vi "CircularBuffer.DVRtoRef.vi"(10 "Ref":T1) -> (2 "Ref":u32 format="%08x")   [LabVIEW 2016, in "CircularBuffer.lvclass"]
doc: "JKI State Machine Objects (SMO) 1.0.0.5\nJKI - JKI\nCopyright (c) 2016, JKI"
uses:
  CircularBuffer.lvclass
  Typedefs/PrivateData--Ref.ctl
  Typedefs/PrivateData--Cluster.ctl
  Typedefs/PublicEvents--Cluster.ctl
  Typedefs/ValueChanged--EventData--Cluster.ctl
  Typedefs/ProtectedEvents--Cluster.ctl
  Typedefs/NewBufferSize--Cluster.ctl
  Typedefs/PrivateEvents--Cluster.ctl
  Typedefs/PrivateEvents--CircularBuffer.GetElement.ctl
  Typedefs/PrivateEvents--CircularBuffer.Initialize.ctl
  types/type/type.lvclass
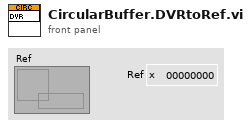
[diagram p1: front panel]
types:
  T1 = typedef "CircularBuffer.lvclass/PrivateData--Ref.ctl" = refnum<data-value>
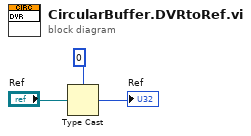
[diagram p0: block diagram]
diagram:
  n1 = Type Cast(type=u32 0 ("Ref"), x="Ref") -> (*(type *) &x=→"Ref":u32)
